vi "lsl destroy outlet.vi"(8 "error in (no error)":errorcluster, 11 "outlet":T1) -> (0 "error out":errorcluster)   [LabVIEW 2018, in "liblsl-LabVIEW.lvlib"]
doc: "extern LIBLSL_C_API void lsl_destroy_outlet(lsl_outlet out);"
uses:
  <userlib>/liblsl-LabVIEW/liblsl-LabVIEW.lvlib
  <userlib>/liblsl-LabVIEW/Custom Controls/lsl_outlet.ctl
  <userlib>/liblsl-LabVIEW/liblsl64.dll
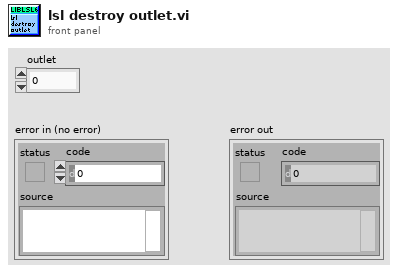
[diagram p1: front panel]
types:
  T1 = typedef "liblsl-LabVIEW.lvlib/lsl_outlet.ctl" = u64
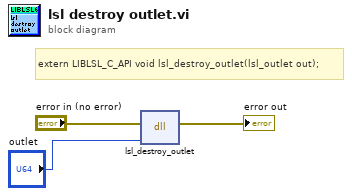
[diagram p0: block diagram]
diagram:
  # "extern LIBLSL_C_API void lsl_destroy_outlet(lsl_outlet out);"
  n1 = dll-call lib="C:/Program Files/National Instruments/LabVIEW 2018/user.lib/liblsl-LabVIEW/liblsl64.dll" fn="lsl_destroy_outlet"(error in="error in (no error)", "out"="outlet") -> (error out=→"error out":errorcluster)  [unwired: 4 in, 1 out]
